vi "Get Registration.vi"(11 "Base Event in":refnum<class "Base Event.lvclass">) -> (2 "Registration":refnum<event-registration>)   [LabVIEW 2021, in "jettl.lvlib" / "Base Event.lvlib" / "Base Event.lvclass"]
uses:
  Base Event.lvclass
  Msg Strategy/Msg Strategy.lvclass
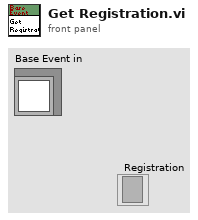
[diagram p1: front panel]
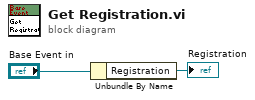
[diagram p0: block diagram]
diagram:
  n1 = Unbundle By Name("Base Event in") -> ("Registration"=→"Registration":refnum<event-registration>)
